vi "HMI Frame.vi"(7 "Expo":dbl(slide) scale=0.0..10.0, 8 "error in (no error)":errorcluster, 11 "ROV in":refnum<class "ROV Host.lvclass">) -> (0 "error out":errorcluster, 3 "ROV out":refnum<class "ROV Host.lvclass">)   [LabVIEW 2012, in "ROV Host.lvclass"]
uses:
  ROV Host.lvclass
  ROV Host.lvclass/ROV Host.ctl
  <vilib>/Utility/inputDevices.llb/joystickAcquire.vi
panel:
  out "direction info":T1
  out "button info":T2
  out "axis info":T3
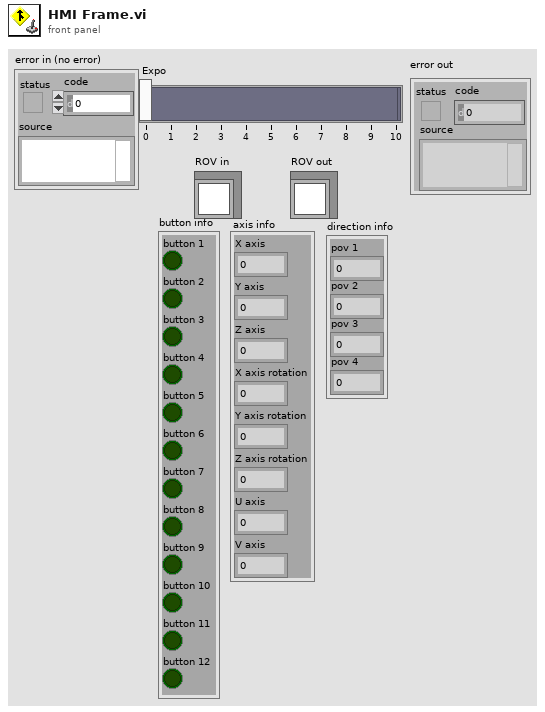
[diagram p1: front panel]
types:
  T1 = cluster{"pov 1":i32, "pov 2":i32, "pov 3":i32, "pov 4":i32}
  T2 = cluster{"button 1":bool, "button 2":bool, "button 3":bool, "button 4":bool, "button 5":bool, "button 6":bool, "button 7":bool, "button 8":bool, "button 9":bool, "button 10":bool, "button 11":bool, "button 12":bool, "button 13":bool, "button 14":bool, "button 15":bool, "button 16":bool, "button 17":bool, "button 18":bool, "button 19":bool, "button 20":bool, "button 21":bool, "button 22":bool, "button 23":bool, "button 24":bool, "button 25":bool, "button 26":bool, "button 27":bool, "button 28":bool, "button 29":bool, "button 30":bool, "button 31":bool, "button 32":bool}
  T3 = cluster{"X axis":i32, "Y axis":i32, "Z axis":i32, "X axis rotation":i32, "Y axis rotation":i32, "Z axis rotation":i32, "U axis":i32, "V axis":i32}
  T4 = typedef "NI_Robotics_Steering Class Types.lvlib/Mecanum Steering Frame.ctl" = refnum<class "NI_Robotics_Mecanum Steering Frame.lvclass">
  T5 = typedef "NI_Robotics_Steering Class Types.lvlib/Differential Steering Frame.ctl" = refnum<class "NI_Robotics_Differential Steering Frame.lvclass">
  T6 = cluster{"mecanum steering frame out":T4, "differential steering frame out":T5}
  T7 = cluster{"device ID":refnum<k1>, "Device Name":string, "axis info":cluster{"X axis":dbl[], "Y axis":dbl[], "Z axis":dbl[], "X axis rotation":dbl[], "Y axis rotation":dbl[], "Z axis rotation":dbl[], "U axis":dbl[], "V axis":dbl[]}}
  T8 = cluster{"button info":cluster{"button 1":bool, "button 2":bool, "button 3":bool, "button 4":bool, "button 5":bool, "button 6":bool, "button 7":bool, "button 8":bool, "button 9":bool, "button 10":bool, "button 11":bool, "button 12":bool, "button 13":bool, "button 14":bool, "button 15":bool, "button 16":bool, "button 17":bool, "button 18":bool, "button 19":bool, "button 20":bool, "button 21":bool, "button 22":bool, "button 23":bool, "button 24":bool, "button 25":bool, "button 26":bool, "button 27":bool, "button 28":bool, "button 29":bool, "button 30":bool, "button 31":bool, "button 32":bool}, "direction info":cluster{"pov 1":i32, "pov 2":i32, "pov 3":i32, "pov 4":i32}, "axis info":cluster{"X axis":i32, "Y axis":i32, "Z axis":i32, "X axis rotation":i32, "Y axis rotation":i32, "Z axis rotation":i32, "U axis":i32, "V axis":i32}}
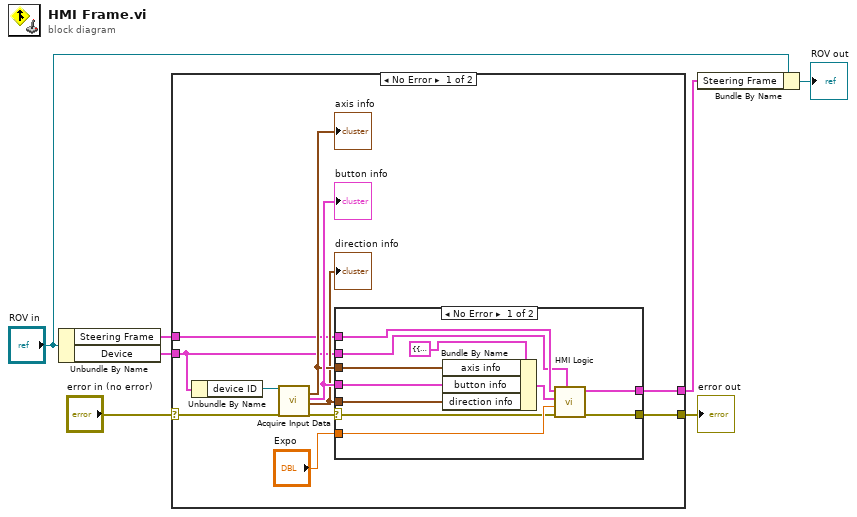
[diagram p0: block diagram]
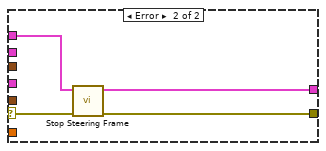
[diagram p2: hidden frame]
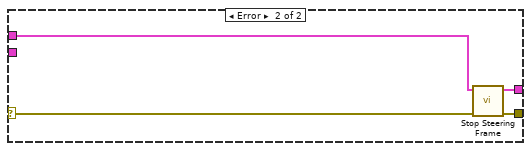
[diagram p3: hidden frame]
diagram:
  n1 = Unbundle By Name("ROV in") -> ("Steering Frame"=w5:T6, "Device"=w4:T7)
  n2 = case shown="No Error" "error in (no error)" {
    selector: "error in (no error)" -> [w11 w35]
    tunnel: [w10 w37] -> w7
    tunnel: w4 -> [w13 _]
    tunnel: w5 -> [w12 w34]
    tunnel: [w9 w36] -> w1
    frame No Error {
      n3 = Unbundle By Name(w13) -> ("device ID"=w17:refnum<k1>)
      n4 = call-poly <vilib>:"Acquire Input Data.vi"("device ID"=w17, "error in (no error)"=w11) -> ("axis info"=w15:T3, "button info"=w16:T2, "direction info"=w14:T1, "error out"=w18:errorcluster)  [unwired: 13 in, 1 out]
      "axis info" <- w15
      "direction info" <- w14
      "button info" <- w16
      n5 = case shown="No Error" w18 {
        selector: w18 -> [w27 w33]
        tunnel: w16 -> [w21 _]
        tunnel: w15 -> [w20 _]
        tunnel: w14 -> [w19 _]
        tunnel: w13 -> [w22 _]
        tunnel: w12 -> [w28 w32]
        tunnel: [w25 w30] -> w10
        tunnel: [w26 w31] -> w9
        tunnel: "Expo" -> [w29 _]
        frame No Error {
          n6 = Bundle By Name(cluster=T8 {"button info"={"button 1"=FALSE, "button 2"=FALSE, "button 3"=FALSE, "button 4"=FALSE, "button 5"=FALSE, "button 6"=FALSE, "button 7"=FALSE, "button 8"=FALSE, "button 9"=FALSE, "button 10"=FALSE, "button 11"=FALSE, "button 12"=FALSE, "button 13"=FALSE, "button 14"=FALSE, "button 15"=FALSE, "button 16"=FALSE, "button 17"=FALSE, "button 18"=FALSE, "button 19"=FALSE, "button 20"=FALSE, "button 21"=FALSE, "button 22"=FALSE, "button 23"=FALSE, "button 24"=FALSE, "button 25"=FALSE, "button 26"=FALSE, "button 27"=FALSE, "button 28"=FALSE, "button 29"=FALSE, "button 30"=FALSE, "button 31"=FALSE, "button 32"=FALSE}, "direction info"={"pov 1"=-1, "pov 2"=-1, "pov 3"=-1, "pov 4"=-1}, "axis info"={"X axis"=3832, "Y axis"=898, "Z axis"=0, "X axis rotation"=-443, "Y axis rotation"=465, "Z axis rotation"=0, "U axis"=0, "V axis"=0}} ("HMI"), "axis info"=w20, "button info"=w21, "direction info"=w19) -> (w24:T8)
          n7 = call "HMI Logic.vi"("Device"=w22, "error in (no error)"=w27, "Expo"=w29, "HMI"=w24, "Steering Frame in"=w28) -> ("error out"=w25:errorcluster, "Steering Frame out"=w26:T6)  [unwired: 5 in]
        }
        frame Error {
          n8 = call "Stop Steering Frame.vi"("error in (no error)"=w33, "Steering Frame in"=w32) -> ("error out"=w30:errorcluster, "Steering Frame out"=w31:T6)  [unwired: 8 in]
        }
      }
    }
    frame Error {
      n9 = call "Stop Steering Frame.vi"("error in (no error)"=w35, "Steering Frame in"=w34) -> ("error out"=w37:errorcluster, "Steering Frame out"=w36:T6)  [unwired: 8 in]
    }
  }
  "error out" <- w7
  n10 = Bundle By Name(cluster="ROV in", "Steering Frame"=w1) -> (→"ROV out":refnum<class "ROV Host.lvclass">)
